vi "Main Program.vi"() -> ()   [LabVIEW 2018]
uses:
  <vilib>/Utility/file.llb/Write Delimited Spreadsheet (string).vi
panel:
  in  "GPIB addess":string="0:17"
  in  "Array":T1(array[cluster])
  out "Area (m^2)":dbl
  in  "Thickness (mm)":dbl format="%#_13g"
  in  "Diameter (mm)":dbl format="%#_13g"
  in  "VISA resource name":refnum<visa-resource-name>
  out "Freq":dbl[](array[numeric])
  out "Loss":cluster{"Y":dbl[], "Y":dbl[]}[](graph)
  out "Permittivity":cluster{"Y":dbl[], "Y":dbl[]}[](graph)
  in  "stop":bool
  in  "# Steps/Decade":i32
  in  "Max Frequency":i32 format="%.0e"
  in  "Min Frequency":i32 format="%.0e"
  in  "Filename":string
  in  "Folder":path
  # "Plot?"
  # "Temp [C]"
  # "Freq. [Hz]"
  # "Cap. [F]"
  # "Perm."
  # "Tan(d)"
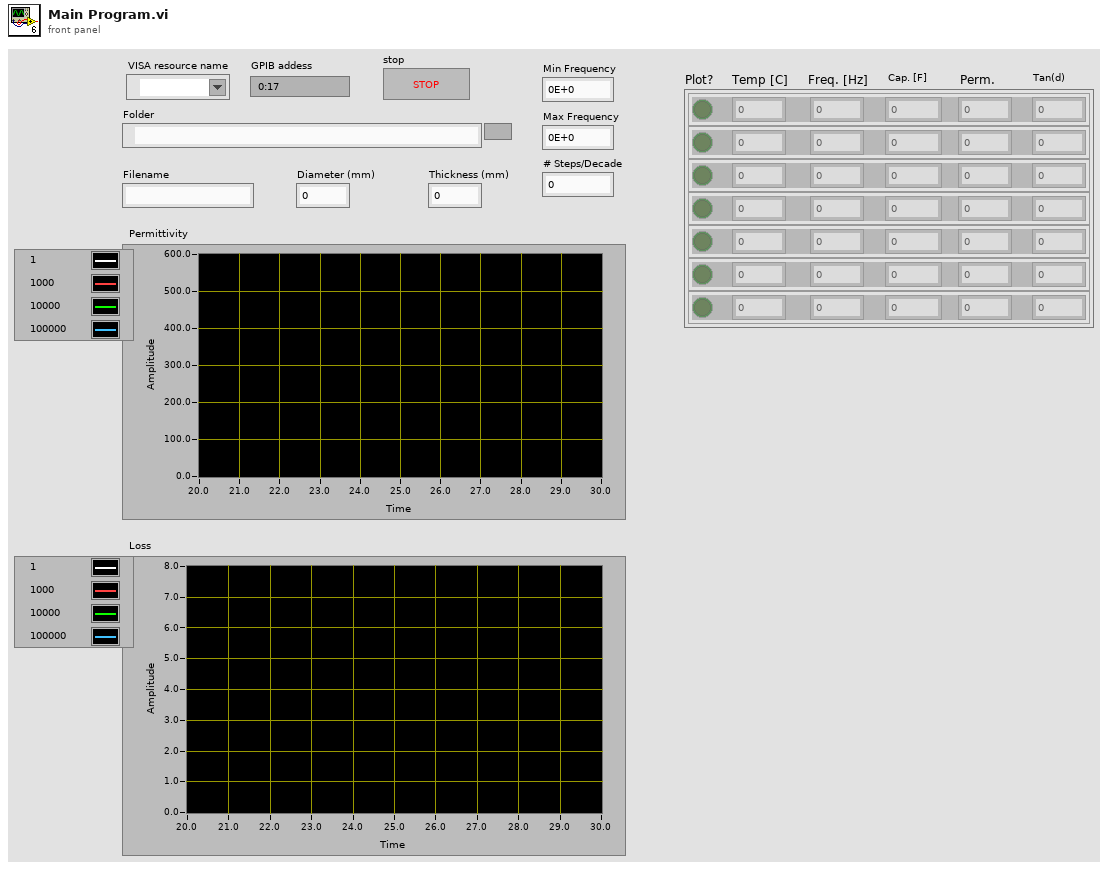
[diagram p1: front panel]
types:
  T1 = cluster{"Plot?":bool, "Temperature":ext, "Capacitance":ext, "Frequency":ext, "Loss":ext, "Permittivity":ext}[]
  T2 = cluster{"Plot?":bool, "Temperature":ext, "Capacitance":ext, "Frequency":ext, "Loss":ext, "Permittivity":ext}
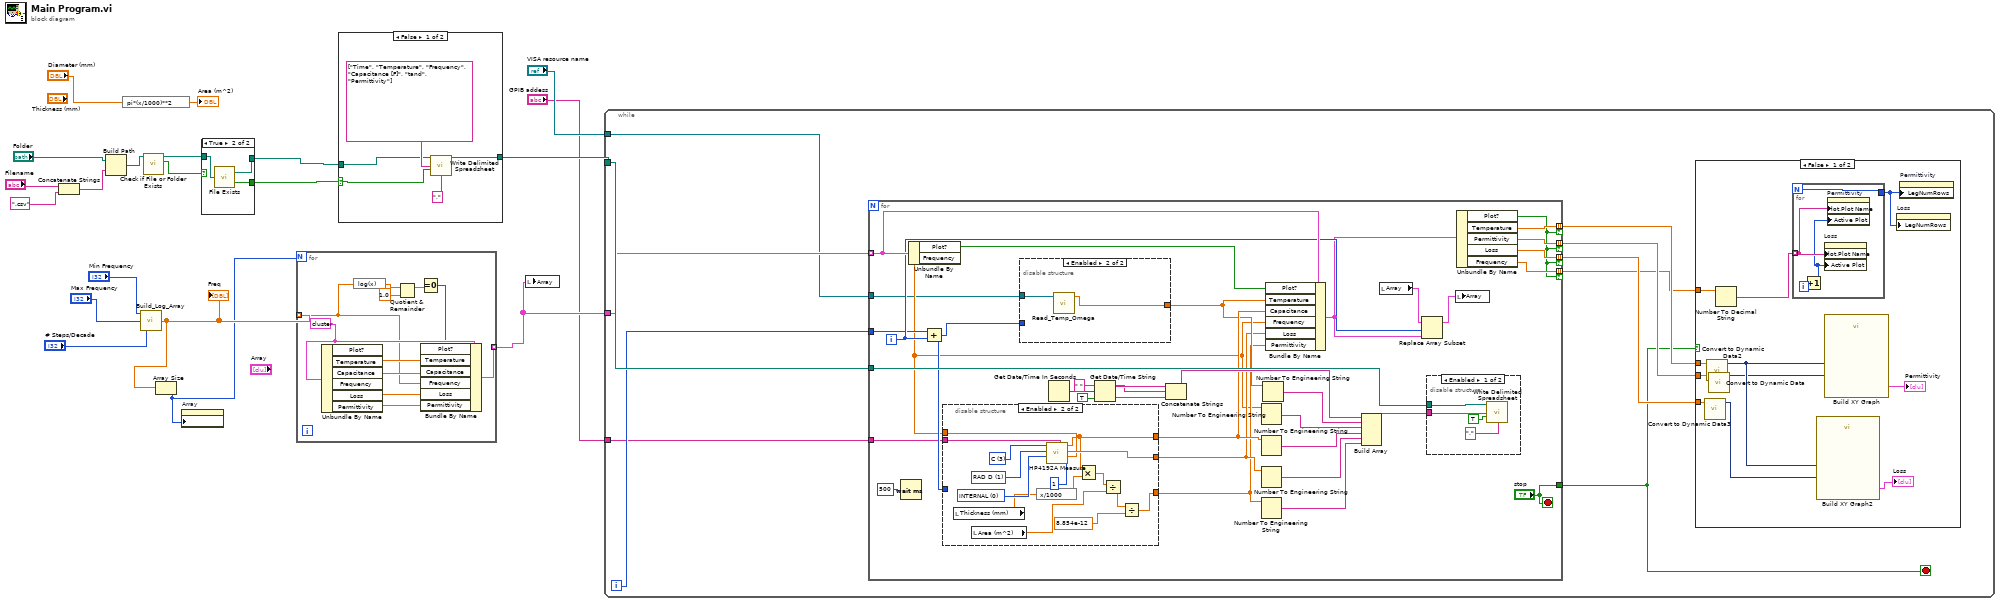
[diagram p0: block diagram]
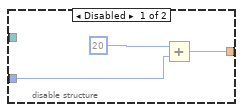
[diagram p3: hidden frame]
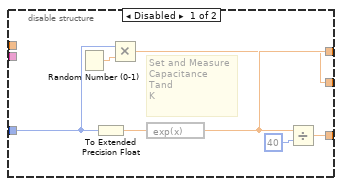
[diagram p4: hidden frame]
diagram:
  n1 = Concatenate Strings("Filename", ".csv") -> (w18:string)
  n2 = Build Path(base path="Folder", name or relative path=w18) -> (appended path=w16:path)
  n3 = expression code="pi*(x/1000)**2"("Diameter (mm)") -> (→"Area (m^2)":dbl)
  n4 = call "Build_Log_Array.vi"("# Steps"="# Steps/Decade", "Max Frequency"="Max Frequency", "Min Frequency"="Min Frequency") -> ("Array"=w2:dbl[])
  "Freq" <- w2
  n5 = call <vilib>:"Check if File or Folder Exists.vi"("path"=w16) -> ("file or folder exists?"=w15:bool, "dup path"=w14:path)  [unwired: 8 in, 1 out]
  n6 = Array Size(array=w2) -> (size(s)=w1:i32)
  n7 = property on="Array" class="Arr (strict)"("Number of Rows"=w1) -> ()  [unwired: 2 in, 2 out]
  n8 = case shown="True" w15 {
    selector: w15 -> [w21 _]
    tunnel: w14 -> [w22 w25]
    tunnel: [w22 w24] -> w9
    tunnel: [w21 w23] -> w8
    frame False {
    }
    frame True {
      n9 = call "File Exists.vi"("Path In"=w25) -> ("Path Out"=w24:path, "Append?"=w23:bool)
    }
  }
  n10 = for {
    N: w1 -> [_]
    tunnel: w2 -> [w30] mode=indexing
    tunnel: [w32] -> w7 mode=indexing
    w31 = T2 {"Plot?"=TRUE, "Temperature"=23.0, "Capacitance"=20.085536923187668, "Frequency"=1.0, "Loss"=2.7981803942322134, "Permittivity"=0.5021384230796917} ("Array")
    n11 = Unbundle By Name(w31) -> ("Temperature"=w36:ext, "Capacitance"=w35:ext, "Loss"=w34:ext, "Permittivity"=w33:ext)  [unwired: 2 out]
    n12 = expression code="log(x)"(w30) -> (w29:dbl)
    n13 = Quotient & Remainder(x=w29, y=1.0) -> (x-y*floor(x/y)=w27:dbl)  [unwired: 1 out]
    n14 = Equal To 0?(x=w27) -> (x = 0?=w26:bool)
    n15 = Bundle By Name(cluster=w31, "Plot?"=w26, "Temperature"=w36, "Capacitance"=w35, "Frequency"=w30, "Loss"=w34, "Permittivity"=w33) -> (w32:T2)
  }
  n16 = case shown="False" w8 {
    selector: w8 -> [w37 _]
    tunnel: [w39 w42] -> w10
    tunnel: w9 -> [w38 w42]
    frame False {
      n17 = call-poly <vilib>:"Write Delimited Spreadsheet.vi"("file path (dialog if empty)"=w38, "1D data"=string[] ["Time", "Temperature", "Frequency", "Capacitance [F]", "tand", "Permittivity"], "append to file? (new file:F)"=w37, "delimiter (\\t)"="," ("delimiter (\\t)")) -> ("new file path (Not A Path if cancelled)"=w39:path)  [unwired: 10 in, 1 out]
    }
    frame True {
    }
  }
  n18 = local write "Array"(w7) -> ()
  n19 = while {
    tunnel: w10 -> [w52]
    tunnel: w7 -> [w51]
    tunnel: "VISA resource name" -> [w44]
    tunnel: "GPIB addess" -> [w43]
    i -> [w47]
    stop <- w45 stop-if-true
    n20 = for {
      tunnel: w52 -> [w90]
      tunnel: w51 -> [w88] mode=indexing
      tunnel: ["stop"] -> w45
      tunnel: [w78] -> w49 mode=indexing if=w71
      tunnel: [w77] -> w50 mode=indexing if=w71
      tunnel: [w76] -> w48 mode=indexing if=w71
      tunnel: w47 -> [w74]
      tunnel: [w72] -> w46 mode=indexing if=w71
      tunnel: w44 -> [w69]
      tunnel: w43 -> [w68]
      i -> [w83]
      stop <- "stop" stop-if-true
      n21 = Wait (ms)(milliseconds to wait=u32 500) -> ()  [unwired: 1 out]
      n22 = Unbundle By Name(w88) -> ("Plot?"=w73:bool, "Frequency"=w70:ext)
      n23 = Add(x=w74, y=w83) -> (x+y=w75:i32)
      n24 = disable-structure shown="Enabled" {
        disable-tunnel: [w114 w120] -> w89
        disable-tunnel: [w113 w126] -> w86
        disable-tunnel: [w112 w123] -> w85
        disable-tunnel: w75 -> [w111 _]
        disable-tunnel: w70 -> [_ w125]
        disable-tunnel: w68 -> [_ w115]
        frame Disabled {
          # "Set and Measure\nCapacitance\nTand\nK"
          n25 = Random Number (0-1)() -> (number: 0 to 1=w110:dbl)
          n26 = To Extended Precision Float(1:w111) -> (0:w108:ext)
          n27 = Multiply(x=w111, y=w110) -> (x*y=w113:dbl)
          n28 = expression code="exp(x)"(w108) -> (w114:ext)
          n29 = Divide(x=w114, y=40) -> (x/y=w112:ext)
        }
        frame Enabled {
          w128 = i16 1 items=["DEG Q", "RAD D", "         R/G"] ("function B (deg q:0)")
          w127 = i16 3 items=["Z/Y", "R/G", "L", "C"] ("function A (z/y:0)")
          w129 = i16 0 items=["INTERNAL", "EXTERNAL", "HOLD/MANUAL"] ("trigger (internal:0)")
          n30 = local read "Thickness (mm)"() -> (w121:dbl)
          n31 = local read "Area (m^2)"() -> (w117:dbl)
          n32 = expression code="x/1000"(w121) -> (w116:dbl)
          n33 = call "HP4192A Measure.vi"("OSC level (V)"=1, "test signal\nfreq (Hz)"=w125, "GPIB addess"=w115, "trigger (internal:0)"=w129, "function B (deg q:0)"=w128, "function A (z/y:0)"=w127) -> ("display B"=w126:dbl, "display A"=w120:dbl)  [unwired: 4 in]
          n34 = Multiply(x=w120, y=w116) -> (x*y=w119:dbl)
          n35 = Divide(x=w119, y=w117) -> (x/y=w118:dbl)
          n36 = Divide(x=w118, y=8.854e-12) -> (x/y=w123:dbl)
        }
      }
      n37 = disable-structure shown="Enabled" {
        disable-tunnel: [w104 w107] -> w87
        disable-tunnel: w75 -> [w103 _]
        disable-tunnel: w69 -> [_ w106]
        frame Disabled {
          n38 = Add(x=20, y=w103) -> (x+y=w104:i32)
        }
        frame Enabled {
          n39 = call "Read_Temp_Omega.vi"("VISA Omega (Serial - COM1)"=w106) -> ("Temperature"=w107:dbl)  [unwired: 9 in, 1 out]
        }
      }
      n40 = Get Date/Time In Seconds() -> (seconds since 1Jan1904=w102:timestamp)
      n41 = Get Date/Time String(seconds (now)=w102, want seconds? (F)=TRUE) -> (date string=w100:string, time string=w99:string)  [unwired: 1 in]
      n42 = Concatenate Strings(w100, " " ("string"), w99) -> (w97:string)
      n43 = Number To Engineering String(4:w70) -> (0:w95:string)  [unwired: 3 in]
      n44 = Number To Engineering String(4:w89) -> (0:w94:string)  [unwired: 3 in]
      n45 = Number To Engineering String(4:w86) -> (0:w93:string)  [unwired: 3 in]
      n46 = Number To Engineering String(4:w85) -> (0:w92:string)  [unwired: 3 in]
      n47 = Number To Engineering String(4:w87) -> (0:w96:string)  [unwired: 3 in]
      n48 = Bundle By Name(cluster=w88, "Plot?"=w73, "Temperature"=w87, "Capacitance"=w89, "Frequency"=w70, "Loss"=w86, "Permittivity"=w85) -> (w79:T2)
      n49 = Build Array(w97, w96, w95, w94, w93, w92) -> (w91:string[])
      n50 = local read "Array"() -> (w82:T1)
      n51 = Replace Array Subset(array=w82, new element=w79, index=w83) -> (w84:T1)
      n52 = disable-structure shown="Enabled" {
        disable-tunnel: w91 -> [w133 _]
        disable-tunnel: w90 -> [w131 _]
        frame Enabled {
          n53 = call-poly <vilib>:"Write Delimited Spreadsheet.vi"("file path (dialog if empty)"=w131, "1D data"=w133, "append to file? (new file:F)"=TRUE ("transpose? (no:F)"), "delimiter (\\t)"="," ("delimiter (\\t)")) -> ()  [unwired: 10 in, 2 out]
        }
        frame Disabled {
        }
      }
      n54 = local write "Array"(w84) -> ()
      n55 = Unbundle By Name(w79) -> ("Plot?"=w71:bool, "Temperature"=w78:ext, "Permittivity"=w77:ext, "Loss"=w76:ext, "Frequency"=w72:ext)
    }
    n56 = case shown="False" w45 {
      tunnel: w50 -> [w62 _]
      tunnel: w49 -> [w61 _]
      tunnel: w48 -> [w58 _]
      tunnel: w46 -> [w54 _]
      frame False {
        n57 = call "Convert to Dynamic Data3"("Array"=w58) -> ("Dynamic Data Type"=w57:dynamicdata)  [unwired: 3 in]
        n58 = call "Convert to Dynamic Data2"("Array"=w61) -> ("Dynamic Data Type"=w59:dynamicdata)  [unwired: 3 in]
        n59 = call "Convert to Dynamic Data"("Array"=w62) -> ("Dynamic Data Type"=w56:dynamicdata)  [unwired: 3 in]
        n60 = Number To Decimal String(number=w54) -> (decimal integer string=w55:string[])  [unwired: 1 in]
        n61 = for {
          N -> [w65]
          tunnel: w55 -> [w67] mode=indexing
          tunnel: [w65] -> w53
          i -> [w66]
          n62 = Increment(x=w66) -> (x+1=w64:i32)
          n63 = property on="Loss" class="XYGraph (strict)"("Plot.Plot Name"=w67, "Active Plot"=w64) -> ()  [unwired: 2 in, 2 out]
          n64 = property on="Permittivity" class="XYGraph (strict)"("Plot.Plot Name"=w67, "Active Plot"=w64) -> ()  [unwired: 2 in, 2 out]
        }
        n65 = call "Build XY Graph2"("Y Input"=w57, "X Input"=w59) -> ("XY Graph"=→"Loss":cluster{"X":dbl[], "Y":dbl[]}[])  [unwired: 8 in, 1 out]
        n66 = call "Build XY Graph"("Y Input"=w56, "X Input"=w59) -> ("XY Graph"=→"Permittivity":cluster{"X":dbl[], "Y":dbl[]}[])  [unwired: 8 in, 1 out]
        n67 = property on="Loss" class="XYGraph (strict)"("LegNumRows"=w53) -> ()  [unwired: 2 in, 2 out]
        n68 = property on="Permittivity" class="XYGraph (strict)"("LegNumRows"=w53) -> ()  [unwired: 2 in, 2 out]
      }
      frame True {
      }
    }
  }
